vi "VI Server_TREE_ActiveCell_ItemName_SET.vi"(4 "Text":string, 6 "AciveCell.Position":T1={"Row Number\n(-2-all clmns)"=0, "Column Number\n(-2 - whole row)"=3} {"Column Number\n(-2 - whole row)" min=-2}, 7 "Label":string, 8 "error in":errorcluster, 9 "Tree.Ref":refnum<vi>, 10 "SingleInstance":bool=TRUE, 11 "VI Server.RefsCluster":T2) -> (0 "error out":errorcluster, 1 "Tree.Ref.DUP":refnum<vi>, 3 "VI Server.RefsCluster.DUP":T2)   [LabVIEW 2020]
uses:
  VI Server_TypeDefs/VI Server_RefsCluster.ctl
  VI Server_TypeDefs/VI Server_TREE_ActiveCell_Pos.ctl
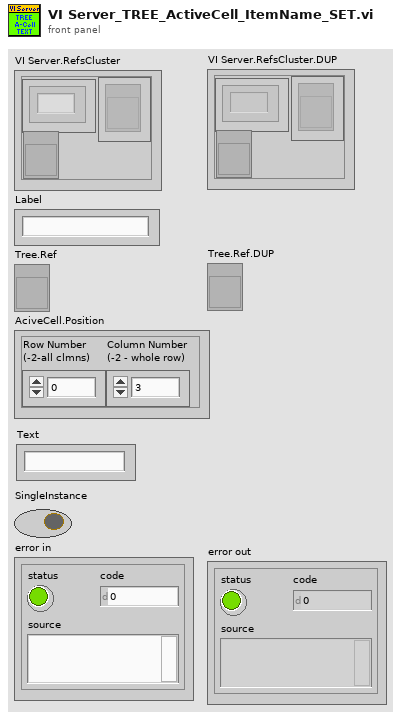
[diagram p1: front panel]
types:
  T1 = typedef "VI Server_TREE_ActiveCell_Pos.ctl" = cluster{"Row Number\n(-2-all clmns)":i32, "Column Number\n(-2 - whole row)":i32}
  T2 = typedef "VI Server_RefsCluster.ctl" = cluster{"Labels":string[], "Refs":refnum<vi>[], "VI Ref":refnum<vi>}
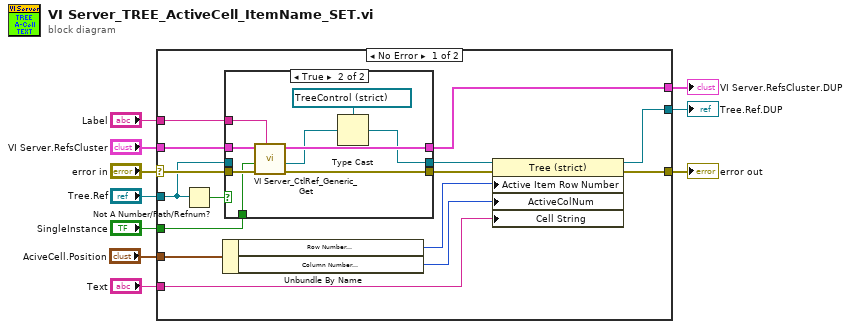
[diagram p0: block diagram]
diagram:
  n1 = case shown="No Error" "error in" {
    selector: "error in" -> [w25 w39]
    tunnel: [w16 w39] -> w9
    tunnel: "VI Server.RefsCluster" -> [w24 w38]
    tunnel: [w23 w38] -> w7
    tunnel: "Label" -> [w22 _]
    tunnel: "SingleInstance" -> [w21 _]
    tunnel: [w15 _] -> w4
    tunnel: "Tree.Ref" -> [w19 _]
    tunnel: "Text" -> [w11 _]
    tunnel: "AciveCell.Position" -> [w14 _]
    frame No Error {
      n2 = Not A Number/Path/Refnum?(number/path/refnum=w19) -> (NaN/Path/Refnum?=w20:bool)
      n3 = Unbundle By Name(w14) -> ("Row Number\n(-2-all clmns)"=w13:i32, "Column Number\n(-2 - whole row)"=w12:i32)
      n4 = case shown="True" w20 {
        tunnel: w25 -> [w28 w37]
        tunnel: w24 -> [w26 w36]
        tunnel: [w26 w35] -> w23
        tunnel: w22 -> [_ w34]
        tunnel: w21 -> [_ w32]
        tunnel: [w27 w30] -> w18
        tunnel: [w28 w29] -> w17
        tunnel: w19 -> [w27 _]
        frame False {
        }
        frame True {
          n5 = call "VI Server_CtlRef_Generic_Get.vi"("Control.Label"=w34, "error in"=w37, "SingleInstance"=w32, "VI Server.RefsCluster"=w36) -> ("error out"=w29:errorcluster, "Control.Ref.Generic"=w33:refnum<vi>, "VI Server.RefsCluster.DUP"=w35:T2)  [unwired: 5 in]
          n6 = Type Cast(type=refnum<vi> refnum ("Tree"), x=w33) -> (*(type *) &x=w30:refnum<vi>)
        }
      }
      n7 = property on="Property Node" class="Tree (strict)"(reference=w18, error in=w17, "Active Item Row Number"=w13, "ActiveColNum"=w12, "Cell String"=w11) -> (reference out=w15:refnum<vi>, error out=w16:errorcluster)
    }
    frame Error {
    }
  }
  "VI Server.RefsCluster.DUP" <- w7
  "error out" <- w9
  "Tree.Ref.DUP" <- w4
